vi "Drive_to_Grid.vi"(1 "Timeout (ms)":dbl, 2 "Distance from Target (m)":dbl, 3 "Speed (m/s)":dbl) -> ()   [LabVIEW 2020]
uses:
  <vilib>/Rock Robotics/WPI/ThirdParty/REV Robotics/REVLib/Typedef/Spark MAX Control Type.ctl
  <vilib>/Rock Robotics/WPI/DriverStation/WPI_DriverStationAllianceInfo.ctl
  Robot Global Data.vi
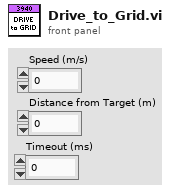
[diagram p1: front panel]
types:
  T1 = typedef "WPI_DriverStationAllianceInfo.ctl" = enum16{"Red", "Blue", "Invalid"}
  T2 = typedef "Spark MAX Control Type.ctl" = enum16{"Percent VBus", "Voltage", "Velocity", "Position", "Smart Motion", "Current", "Smart Velocity"}
  T3 = cluster{"P Gain":dbl, "I Gain":dbl, "D Gain":dbl, "F Gain":dbl, "I Zone":dbl, "Min Output":dbl, "Max Output":dbl}
  T4 = typedef "WPI_MotorControlDeviceRef.ctl" = cluster{"DeviceStatus":errorcluster, "Type":T5, "PWM":cluster{"PWM Channel":T6, "DeadBand":T7}, "CAN":cluster{"Device Number":u8, "SetOutput VI Ref":variant, "GetOutput VI Ref":variant, "Enable VI Ref":variant, "Disable VI Ref":variant, "Data":variant}, "Invert":bool, "DIO PWM":cluster{"PWM \"Enable\" Channel":T6, "DIOChannel":T8, "PWM Rate":dbl}}
  T5 = typedef "WPI_MotorControlType.ctl" = enum16{"PWM", "CAN", "DIO PWM"}
  T6 = typedef "FPGA_DIOPWMChannel.ctl" = enum8{"PWM 0", "PWM 1", "PWM 2", "PWM 3", "PWM 4", "PWM 5", "PWM 6", "PWM 7", "PWM 8", "PWM 9", "PWM MXP 0", "PWM MXP 1", "PWM MXP 2", "PWM MXP 3", "PWM MXP 4", "PWM MXP 5", "PWM MXP 6", "PWM MXP 7", "PWM MXP 8", "PWM MXP 9", "Invalid"}
  T7 = typedef "WPI_PWMDeadband.ctl" = cluster{"Name":string, "maxPositivePwm":i32, "minPositivePwm":i32, "centerPwm":i32, "maxNegativePwm":i32, "minNegativePwm":i32, "angularRange":u16}
  T8 = typedef "FPGA_DIOChannel.ctl" = enum8{"DIO 0", "DIO 1", "DIO 2", "DIO 3", "DIO 4", "DIO 5", "DIO 6", "DIO 7", "DIO 8", "DIO 9", "DIO MXP 0", "DIO MXP 1", "DIO MXP 2", "DIO MXP 3", "DIO MXP 4", "DIO MXP 5", "DIO MXP 6", "DIO MXP 7", "DIO MXP 8", "DIO MXP 9", "DIO MXP 10", "DIO MXP 11", "DIO MXP 12", "DIO MXP 13", "DIO MXP 14", "DIO MXP 15", "SPI Port CS1", "SPI Port CS2", "SPI Port CS3", "SPI Port MISO", "SPI Port MOSI", "Invalid"}
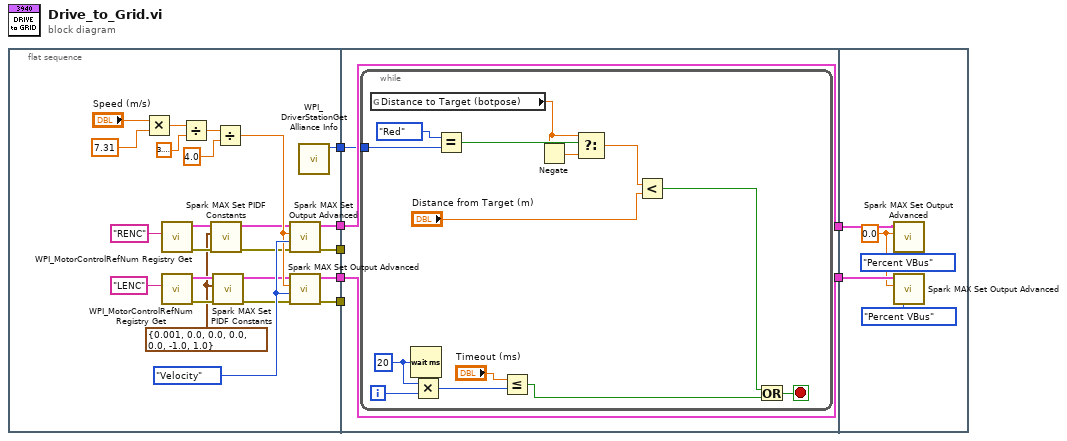
[diagram p0: block diagram]
diagram:
  n1 = flat-sequence {
    tunnel: [w17] -> w7
    tunnel: [w16] -> w6
    tunnel: [w15] -> w5
    tunnel: [w14] -> w4
    tunnel: [w8] -> w1
    tunnel: w7 -> [w34]
    tunnel: w6 -> [w33]
    tunnel: w5 -> [_]
    tunnel: w4 -> [_]
    tunnel: [w34] -> w3
    tunnel: [w33] -> w2
    tunnel: w1 -> [w32]
    tunnel: w3 -> [w53]
    tunnel: w2 -> [w52]
    frame #0 {
      w24 = Spark_MAX_Control_Type."Velocity" ("Control Mode")
      w25 = T3 {"P Gain"=0.001, "I Gain"=0.0, "D Gain"=0.0, "F Gain"=0.0, "I Zone"=0.0, "Min Output"=-1.0, "Max Output"=1.0} ("PID Constants")
      n2 = Multiply(x="Speed (m/s)", y=7.31) -> (x*y=w22:dbl)
      n3 = call <vilib>:"WPI_MotorControlRefNum Registry Get.vi"("refnum name"="RENC") -> ("error out"=w29:errorcluster, "MotorControlDevRef"=w28:T4)  [unwired: 9 in]
      n4 = call <vilib>:"WPI_MotorControlRefNum Registry Get.vi"("refnum name"="LENC") -> ("error out"=w27:errorcluster, "MotorControlDevRef"=w26:T4)  [unwired: 9 in]
      n5 = Divide(x=w22, y=3.141592653589793) -> (x/y=w20:dbl)
      n6 = call <vilib>:"Spark MAX Set PIDF Constants.vi"("error in"=w29, "PID Constants"=w25, "MotorControlDeviceRef"=w28) -> ("error out"=w9:errorcluster, "MotorControlDeviceRef"=w12:T4)  [unwired: 7 in]
      n7 = call <vilib>:"Spark MAX Set PIDF Constants.vi"("error in"=w27, "PID Constants"=w25, "MotorControlDeviceRef"=w26) -> ("error out"=w10:errorcluster, "MotorControlDeviceRef"=w11:T4)  [unwired: 7 in]
      n8 = Divide(x=w20, y=4.0) -> (x/y=w18:dbl)
      n9 = call <vilib>:"Spark MAX Set Output Advanced.vi"("error in (no error)"=w9, "Control Mode"=w24, "Setpoint"=w18, "MotorControlDevRef"=w12) -> ("error out"=w14:errorcluster, "MotorControlDevRef"=w17:T4)  [unwired: 6 in]
      n10 = call <vilib>:"Spark MAX Set Output Advanced.vi"("error in (no error)"=w10, "Control Mode"=w24, "Setpoint"=w18, "MotorControlDevRef"=w11) -> ("error out"=w15:errorcluster, "MotorControlDevRef"=w16:T4)  [unwired: 6 in]
      n11 = call <vilib>:"WPI_DriverStationGet Alliance Info.vi"() -> ("Alliance"=w8:T1)  [unwired: 6 in, 5 out]
    }
    frame #1 {
      n12 = while {
        tunnel: w32 -> [w40]
        i -> [w48]
        stop <- w43 stop-if-true
        w47 = u32 20 ("milliseconds to wait")
        n13 = global read "Robot Global Data.vi" "Distance to Target (botpose)"() -> (w38:dbl)
        n14 = Wait (ms)(milliseconds to wait=w47) -> ()  [unwired: 1 out]
        n15 = Multiply(x=w47, y=w48) -> (x*y=w46:u32)
        n16 = Equal?(x=WPI_DriverStationAllianceInfo."Red" ("Alliance"), y=w40) -> (x = y?=w39:bool)
        n17 = Less Or Equal?(x="Timeout (ms)", y=w46) -> (x <= y?=w44:bool)
        n18 = Negate(x=w38) -> (-x=w37:dbl)
        n19 = Select(t=w38, s=w39, f=w37) -> (s? t:f=w35:dbl)
        n20 = Less?(x=w35, y="Distance from Target (m)") -> (x < y?=w42:bool)
        n21 = Or(x=w42, y=w44) -> (x .or. y?=w43:bool)
      }
    }
    frame #2 {
      w51 = 0.0 ("Setpoint")
      n22 = call <vilib>:"Spark MAX Set Output Advanced.vi"("Control Mode"=Spark_MAX_Control_Type."Percent VBus", "Setpoint"=w51, "MotorControlDevRef"=w53) -> ()  [unwired: 7 in, 2 out]
      n23 = call <vilib>:"Spark MAX Set Output Advanced.vi"("Control Mode"=Spark_MAX_Control_Type."Percent VBus", "Setpoint"=w51, "MotorControlDevRef"=w52) -> ()  [unwired: 7 in, 2 out]
    }
  }
